vi "Main.vi"(11 "Module Admin":refnum<class "Delacor_lib_QMH_Cloneable Module Admin.lvclass">) -> ()   [LabVIEW 2024, in "Message.lvlib"]
doc: "This template is based off of the Queued Message Handler design pattern and the Queued Message Handler project template that ships with LabVIEW.\n\nThe main difference is that the queue is private to this module and communication between modules is performed via Broadcast and Request events.\n\nRequest events are wrapped in public API methods and are handled in the Event Handling Loop (EHL) of this VI. Any module can register for Broadcast events sent by this module. The EHL generates messages based on user interface actions.\n\nThe Message Handling Loop (MHL) processes messages generated by the EHL, or by other messages. The messages are string values, so new messages can be added easily to the Message Cases case structure in the MHL. Each message cluster can also provide an optional value for Message Data, which is a variant that can be converted to whatever message-specific data is required.\n_____\nBased on DQMH Dev Tools: Project Template 7.1.0.1503."
uses:
  Message.lvlib
  <vilib>/Delacor/Delacor QMH/Libraries/Cloneable Module Admin_class/Delacor_lib_QMH_Cloneable Module Admin.lvclass
  C:/Program Files (x86)/National Instruments/LabVIEW 2024/vi.lib/Delacor/Delacor QMH/Libraries/Module Admin_class/Delacor_lib_QMH_Module Admin.lvclass
  Module Data--cluster.ctl
  <vilib>/Delacor/Delacor QMH/Libraries/Cloneable Module Admin_class/Delacor_lib_QMH_Cloneable Module Admin.lvclass/Delacor_lib_QMH_Cloneable Module Admin.ctl
  Stop Argument--cluster.ctl
  <vilib>/Delacor/Delacor QMH/Libraries/Message Queue_class/Delacor_lib_QMH_Message Queue.lvclass/Delacor_lib_QMH_Message Queue.ctl
  <vilib>/Delacor/Delacor QMH/Libraries/Module Admin_class/Delacor_lib_QMH_Module Admin.lvclass/Delacor_lib_QMH_Module Admin.ctl
  Draw FP in Subpanel Argument--cluster.ctl
  Remove From Subpanel Argument--cluster.ctl
  Set Message Argument--cluster.ctl
  Append String Argument--cluster.ctl
  Set Text Font Settings Argument--cluster.ctl
  <vilib>/Utility/miscctls.llb/LVFontTypeDef.ctl
  <vilib>/Delacor/Delacor QMH/Libraries/Cloneable Module Admin_class/Delacor_lib_QMH_Get Module ID.vi
  <vilib>/Delacor/Delacor QMH/Libraries/Message Queue_class/Delacor_lib_QMH_Enqueue Message (Single).vi
  <vilib>/Delacor/Delacor QMH/Libraries/Module Admin_class/Delacor_lib_QMH_Get External Launch.vi
  <vilib>/Delacor/Delacor QMH/Libraries/Message Queue_class/Delacor_lib_QMH_Message Queue.lvclass
panel:
  out "Message":string
  out "error out":errorcluster
  out "String":string
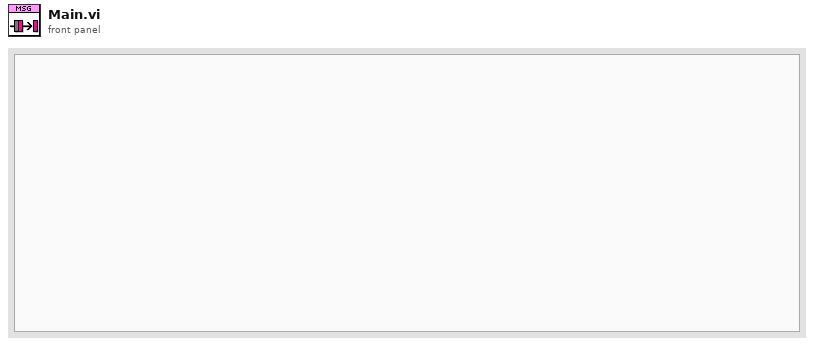
[diagram p1: front panel]
types:
  T1 = typedef "Message.lvlib/Request Events--cluster.ctl" = cluster{"Stop Module":refnum<user-event>, "Show Panel":refnum<user-event>, "Hide Panel":refnum<user-event>, "Show Diagram":refnum<user-event>, "Get Module Execution Status":refnum<user-event>, "Draw FP in Subpanel":refnum<user-event>, "Remove From Subpanel":refnum<user-event>, "Set Message":refnum<user-event>, "Append String":refnum<user-event>, "Set Text Font Settings":refnum<user-event>}
  T2 = typedef "Message.lvlib/Module Data--cluster.ctl" = cluster{"Status":string, "Sub Panel":refnum<vi>, "Message Ref":refnum<vi>}
  T3 = enum32{"invalid lock state", "Not Locked", "Locked (No Password)", "Password-protected"}
  T4 = typedef "Message.lvlib/Stop Argument--cluster.ctl" = cluster{"Module ID":i32, "Origin":string, "Exit via Stop Module Req?":bool, "Wait for Module to stop?":bool}
  T5 = typedef "Message.lvlib/Draw FP in Subpanel Argument--cluster.ctl" = cluster{"Module ID":i32, "Sub Panel":refnum<vi>}
  T6 = typedef "Message.lvlib/Remove From Subpanel Argument--cluster.ctl" = cluster{"Module ID":i32, "Boolean":bool}
  T7 = typedef "Message.lvlib/Set Message Argument--cluster.ctl" = cluster{"Module ID":i32, "Message":string}
  T8 = typedef "Message.lvlib/Append String Argument--cluster.ctl" = cluster{"Module ID":i32, "String":string}
  T9 = typedef "Message.lvlib/Set Text Font Settings Argument--cluster.ctl" = cluster{"Module ID":i32, "Font Settings":cluster{"Text.Font":T10, "Text.Justification":enum16{"Left", "Center", "Right"}}}
  T10 = typedef "LVFontTypeDef.ctl" = cluster{"Font Name":string, "Size":u16, "Bold":bool, "Italic":bool, "Underline":bool, "Strikeout":bool, "Color":u32}
  T11 = enum32{"Invalid", "Standard", "Closed", "Hidden", "Minimized", "Maximized"}
  T12 = cluster{"Text.Font":T10, "Text.Justification":enum16{"Left", "Center", "Right"}}
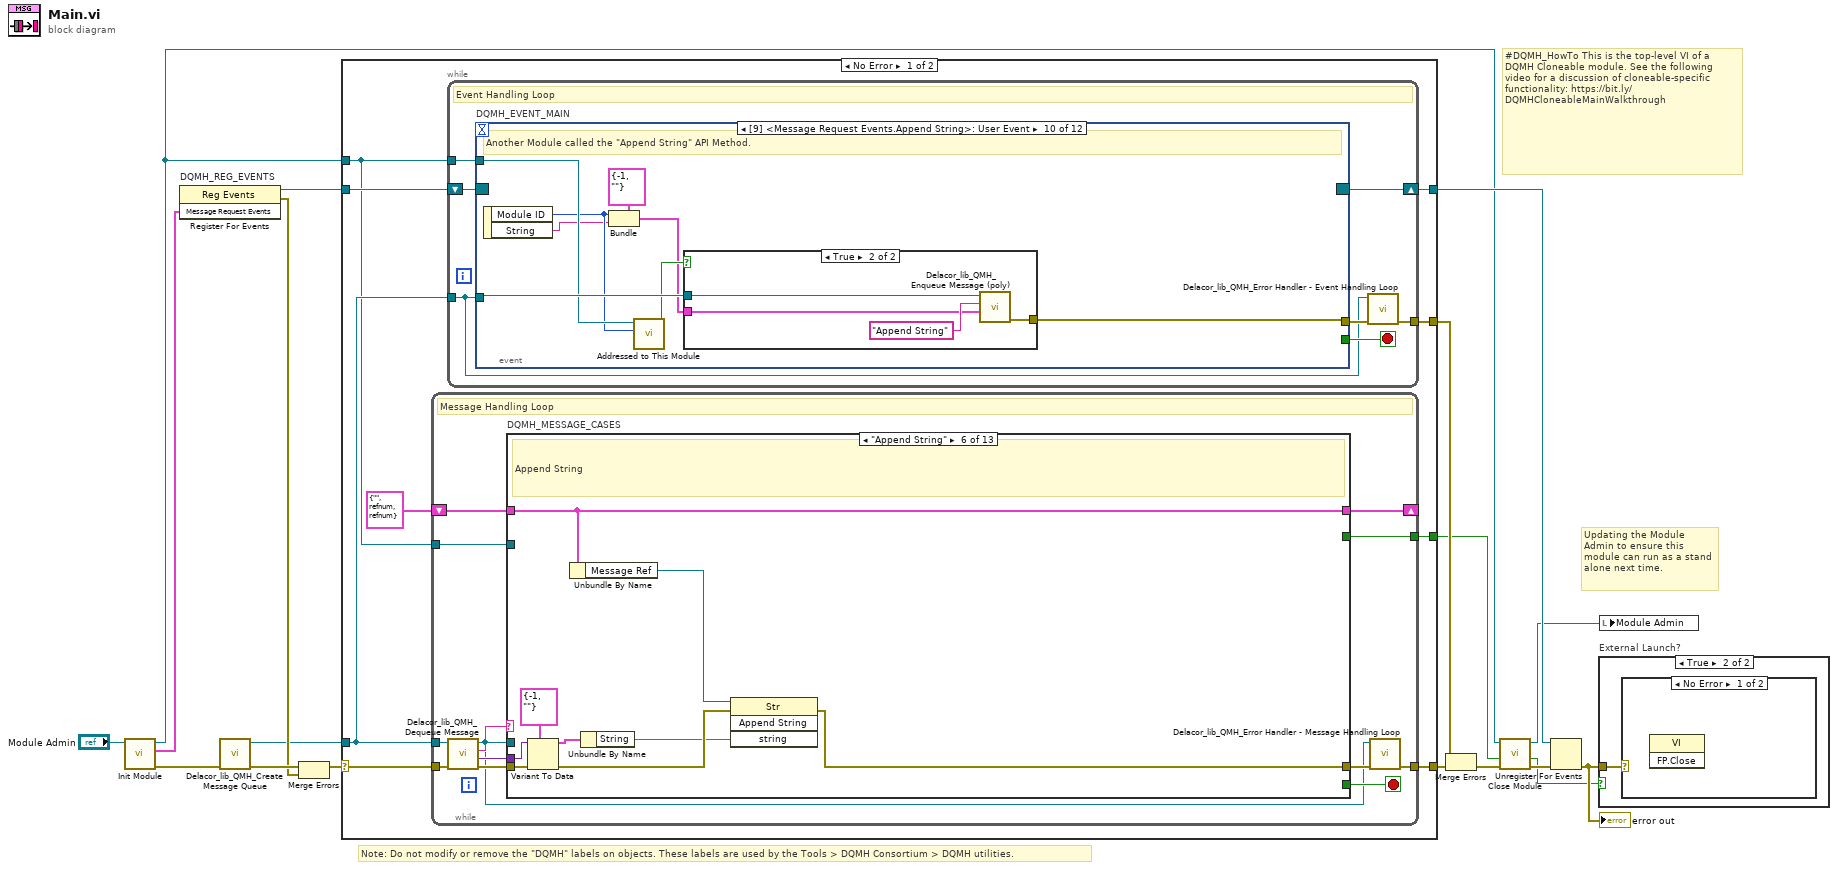
[diagram p0: block diagram]
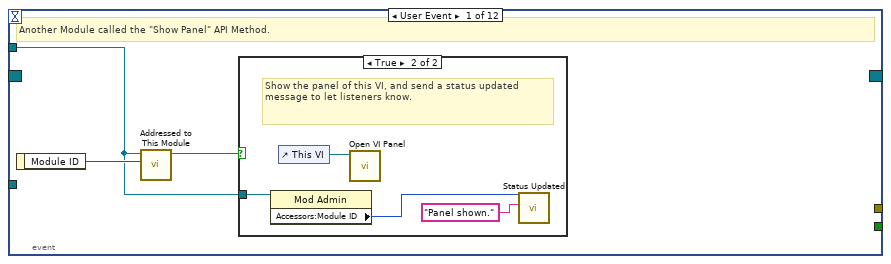
[diagram p2: hidden frame]
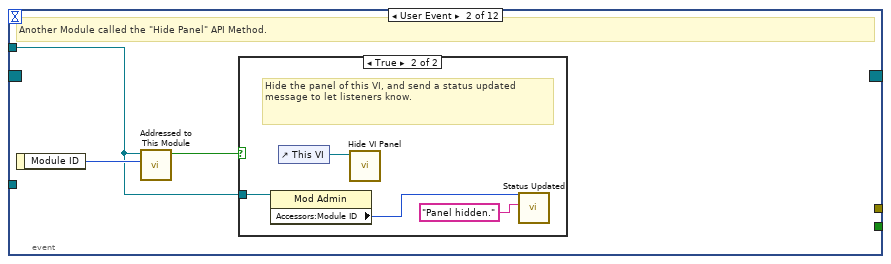
[diagram p4: hidden frame]
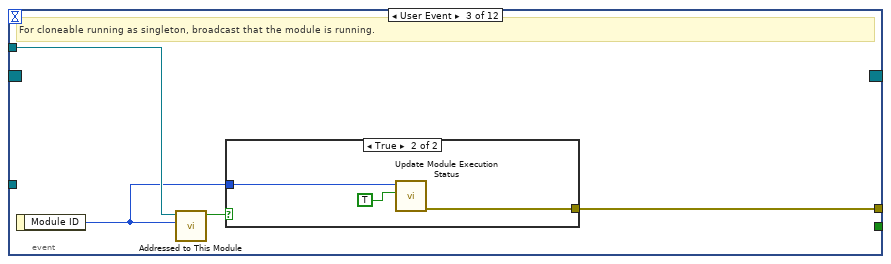
[diagram p6: hidden frame]
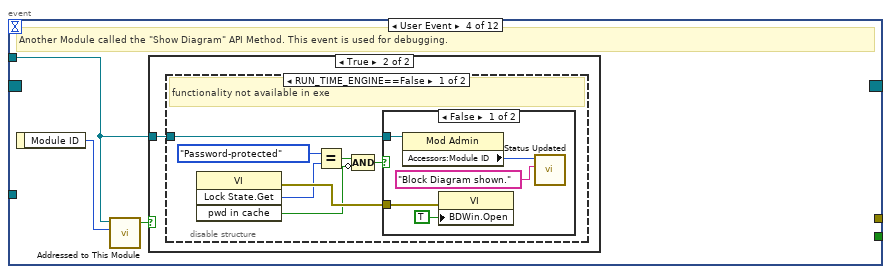
[diagram p8: hidden frame]
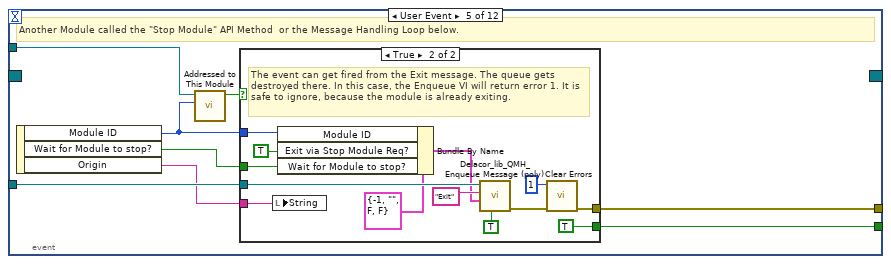
[diagram p12: hidden frame]
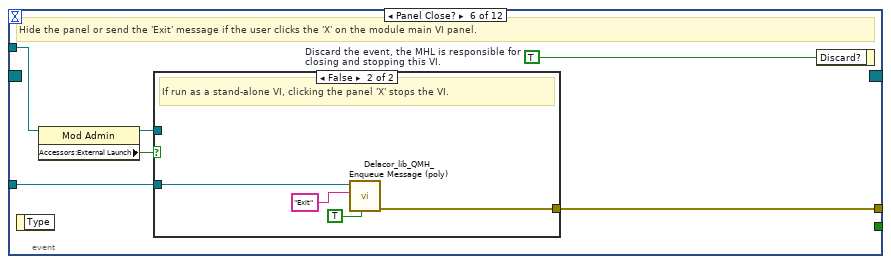
[diagram p14: hidden frame]
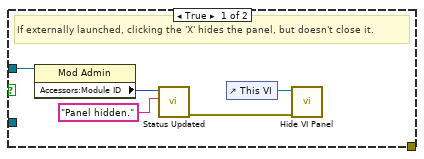
[diagram p15: hidden frame]
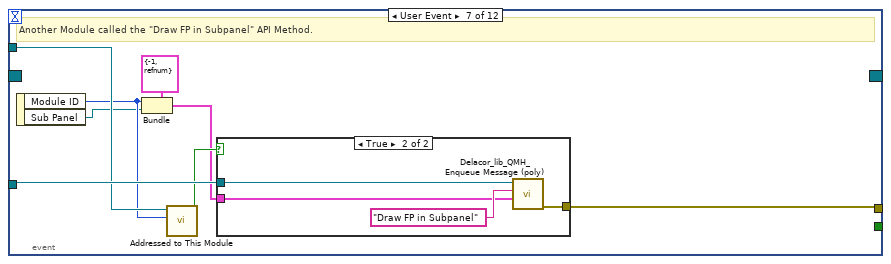
[diagram p16: hidden frame]
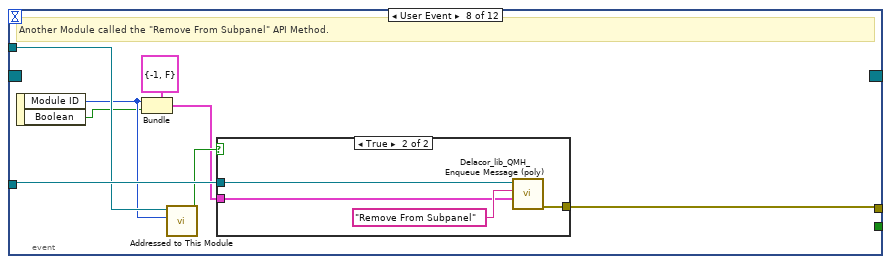
[diagram p18: hidden frame]
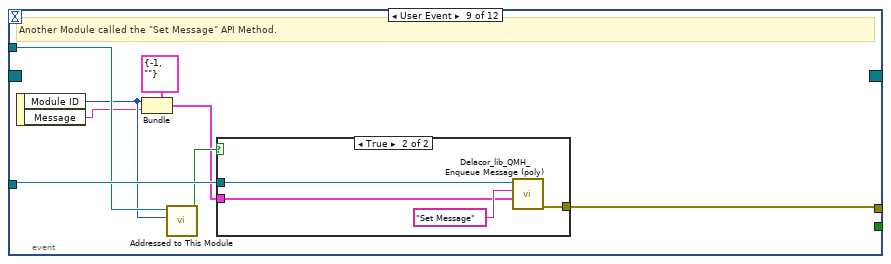
[diagram p20: hidden frame]
diagram:
  # "#DQMH_HowTo This is the top-level VI of a DQMH Cloneable module. See the following video for a discussion of cloneable-specific functionality: https://bit.ly/DQMHCloneableMainWalkthrough"
  # "Note: Do not modify or remove the \"DQMH\" labels on objects. These labels are used by the Tools > DQMH Consortium > DQMH utilities."
  # "Updating the Module Admin to ensure this module can run as a stand alone next time."
  n1 = call "Init Module.vi"("Cloneable Module Admin in"="Module Admin") -> ("error out"=w15:errorcluster, "Message Request Events"=w7:T1, "Cloneable Module Admin out"=w4:refnum<class "Delacor_lib_QMH_Cloneable Module Admin.lvclass">)  [unwired: 8 in]
  n2 = register-events "DQMH_REG_EVENTS"(w7) -> (reference out=w8:refnum<event-registration>, error out=w10:errorcluster)  [unwired: 2 in]
  n3 = call <vilib>:"Delacor_lib_QMH_Create Message Queue.vi"("error in"=w15) -> ("error out"=w12:errorcluster, "Message Queue"=w6:refnum<class "Delacor_lib_QMH_Message Queue.lvclass">)  [unwired: 9 in]
  n4 = Merge Errors(w12, w10) -> (w11:errorcluster)
  n5 = case shown="No Error" w11 {
    selector: w11 -> [w25 w358]
    tunnel: [w27 w357] -> w16
    tunnel: [w24 w356] -> w9
    tunnel: w8 -> [w22 w356]
    tunnel: w6 -> [w21 w349]
    tunnel: [w26 _] -> w17
    tunnel: w4 -> [w20 w352]
    tunnel: [w19 _] -> w2
    frame No Error {
      n6 = while {
        tunnel: w21 -> [w172]
        shift-right: [w179] -> _
        shift-left: T2 {"Status"="", "Sub Panel"=refnum, "Message Ref"=refnum} ("Data Cluster") -> [w180]
        tunnel: w25 -> [w183]
        tunnel: [w181] -> w27
        tunnel: w20 -> [w174]
        tunnel: [w173] -> w19
        stop <- w178 stop-if-true
        # "Message Handling Loop"
        n7 = call-dynamic "Delacor_lib_QMH_Dequeue Message.vi"("error in"=w183, "Message Queue in"=w172) -> ("error out"=w182:errorcluster, "Message Data"=w176:variant, "Message"=w177:string, "Message Queue out"=w175:refnum<class "Delacor_lib_QMH_Message Queue.lvclass">)  [unwired: 6 in]
        n8 = case "DQMH_MESSAGE_CASES" shown="\"Append String\"" w177 {
          selector: w177 -> [_ _ _ _ _ _ _ _ _ _ _ _ w338]
          tunnel: w175 -> [_ _ _ _ _ _ _ _ _ _ w302 w330 _]
          tunnel: w182 -> [w203 w207 w226 w246 w263 w272 w282 w291 w298 w300 w312 w336 w347]
          tunnel: [w201 w207 w222 w244 w262 w265 w275 w287 w297 w300 w308 w331 w348] -> w184
          tunnel: w180 -> [w194 w206 w212 w238 w261 w268 w277 w289 w296 w299 w306 w320 w345]
          tunnel: [w193 w206 w213 w234 w261 w268 w277 w289 w296 w299 w306 w320 w345] -> w179
          tunnel: [_ _ _ _ _ _ _ _ _ _ _ w329 _] -> w178
          tunnel: w176 -> [_ _ w221 w243 w260 w271 w281 w290 _ _ w305 w327 _]
          tunnel: w174 -> [w189 _ w210 w237 w257 _ _ _ _ _ w304 w322 w344]
          tunnel: [_ _ _ _ _ _ _ _ _ _ _ w325 _] -> w173
          frame "Initialize" {
            w186 = "Initial Message" ("Initial Message")
            # "Initialize - Any operation that needs to be done before the module can receive messages. Synchronize Caller Events.vi will inform Start Module.vi that the module has launched and is ready to receive messages. Module Did Init.vi will broadcast that the module initialized."
            n9 = call "Synchronize Caller Events.vi"("error in"=w203, "Module Admin"=w189) -> ("error out"=w202:errorcluster, "Module Admin out"=w188:refnum<class "Delacor_lib_QMH_Cloneable Module Admin.lvclass">)  [unwired: 8 in]
            n10 = property on="Property Node" class="Mod Admin"(reference=w188) -> ("Accessors:Module ID"=w187:i32, "Accessors:External Launch"=w190:bool)  [unwired: 1 in, 2 out]
            n11 = call "Module Name--constant.vi"("Module ID"=w187) -> ("Module Name"=w198:string)  [unwired: 10 in]
            n12 = property on="Property Node" class="VI"("Front Panel.Title"=w198) -> (reference out=w200:refnum<vi>, error out=w205:errorcluster)  [unwired: 2 in]
            n13 = Select(t=T11."Hidden" ("State"), s=w190, f=T11."Standard" ("State")) -> (s? t:f=w195:T11)
            n14 = control-ref of="Message"() -> (w185:refnum<vi>)
            n15 = invoke on="Invoke Node" class="VI" method="FP.Open"(reference=w200, error in=w205, "State"=w195) -> (reference out=w199:refnum<vi>, error out=w204:errorcluster)  [unwired: 2 in, 3 out]
            n16 = Bundle By Name(cluster=w194, "Status"=w186, "Message Ref"=w185) -> (w193:T2)
            n17 = invoke on="Invoke Node" class="VI" method="FP.Center"(reference=w199, error in=w204) -> ()  [unwired: 1 in, 3 out]
            n18 = call "Module Name--constant.vi"("Module ID"=w187) -> ("Module Name"=w191:string)  [unwired: 10 in]
            n19 = call "Module Did Init.vi"("error in"=w202, "Initialized?"=TRUE, "Origin"=w191, "Module ID"=w187) -> ("error out"=w201:errorcluster)  [unwired: 7 in]
            "String" <- w186
          }
          frame "---Module Specific---" {
            # "Separator -- The following cases handle messages specific to this Module."
          }
          frame "Draw FP in Subpanel" {
            # "Draw FP in Subpanel"
            n20 = Variant To Data(error in=w226, type=T5 {"Module ID"=-1, "Sub Panel"=refnum} ("Draw FP in Subpanel Argument"), Variant=w221) -> (data=w219:T5, error out=w223:errorcluster)
            n21 = property class="Mod Admin"(reference=w210) -> ("Accessors:Module ID"=w209:i32)  [unwired: 1 in, 2 out]
            n22 = Unbundle By Name(w219) -> ("Sub Panel"=w211:refnum<vi>)
            n23 = control-ref of="This VI"() -> (w216:refnum<vi>)
            n24 = property class="VI"(reference=w216, error in=w223) -> (reference out=w215:refnum<vi>, error out=w224:errorcluster, "FP.State"=w214:T11)
            n25 = case shown="\"Closed\"" w214 {
              tunnel: [w227 w230] -> w217
              tunnel: [w228 w232] -> w225
              tunnel: w224 -> [w228 w231]
              tunnel: w215 -> [w227 w229]
              frame "Closed" {
              }
              frame "Standard", Default {
                n26 = invoke class="VI" method="FP.Close"(reference=w229, error in=w231) -> (reference out=w230:refnum<vi>, error out=w232:errorcluster)  [unwired: 1 in, 1 out]
              }
            }
            n27 = invoke class="SubPnl" method="Insert VI"(reference=w211, error in=w225, "VI Ref"=w217) -> (reference out=w218:refnum<vi>, error out=w222:errorcluster)  [unwired: 1 in, 2 out]
            n28 = call "Status Updated.vi"("error in"=w222, "Status"="Front Panel Inserted in Subpanel", "Module ID"=w209) -> ()  [unwired: 8 in, 1 out]
            n29 = Bundle By Name(cluster=w212, "Sub Panel"=w218) -> (w213:T2)
          }
          frame "Remove From Subpanel" {
            # "Remove From Subpanel"
            n30 = Variant To Data(error in=w246, type=T6 {"Module ID"=-1, "Boolean"=FALSE} ("Remove From Subpanel Argument"), Variant=w243) -> (data=w241:T6, error out=w245:errorcluster)
            n31 = Unbundle By Name(w241) -> ()  [unwired: 2 out]
            n32 = property class="Mod Admin"(reference=w237) -> ("Accessors:Module ID"=w236:i32)  [unwired: 1 in, 2 out]
            n33 = Unbundle By Name(w238) -> ("Sub Panel"=w240:refnum<vi>)
            n34 = Not A Number/Path/Refnum?(number/path/refnum=w240) -> (NaN/Path/Refnum?=w239:bool)
            n35 = case shown="False" w239 {
              tunnel: w245 -> [w250 w252]
              tunnel: [w249 w252] -> w244
              tunnel: w240 -> [w248 _]
              tunnel: ["Panel Removed from Subpanel" "This module has not been inserted into the subpanel"] -> w235
              frame False {
                n36 = invoke class="SubPnl" method="Remove VI"(reference=w248, error in=w250) -> (error out=w249:errorcluster)  [unwired: 1 in, 2 out]
              }
              frame True {
              }
            }
            n37 = Bundle By Name(cluster=w238, "Sub Panel"=refnum<vi> refnum) -> (w234:T2)
            n38 = call "Status Updated.vi"("error in"=w244, "Status"=w235, "Module ID"=w236) -> ()  [unwired: 8 in, 1 out]
          }
          frame "Set Message" {
            # "Set Message"
            n39 = Variant To Data(error in=w263, type=T7 {"Module ID"=-1, "Message"=""} ("Set Message Argument"), Variant=w260) -> (data=w258:T7, error out=w262:errorcluster)
            n40 = Unbundle By Name(w258) -> ("Message"=w255:string)  [unwired: 1 out]
            "Message" <- w255
            n41 = property class="Mod Admin"(reference=w257) -> ("Accessors:Module ID"=w256:i32)  [unwired: 1 in, 2 out]
            n42 = Format Into String(format string="Message Set to: %s", w255) -> (resulting string=w254:string)  [unwired: 2 in, 1 out]
            n43 = call "Status Updated.vi"("Status"=w254, "Module ID"=w256) -> ()  [unwired: 9 in, 1 out]
          }
          frame "Append String" {
            # "Append String"
            n44 = Variant To Data(error in=w272, type=T8 {"Module ID"=-1, "String"=""} ("Append String Argument"), Variant=w271) -> (data=w269:T8, error out=w266:errorcluster)
            n45 = Unbundle By Name(w268) -> ("Message Ref"=w267:refnum<vi>)
            n46 = Unbundle By Name(w269) -> ("String"=w264:string)
            n47 = invoke class="Str" method="Append String"(reference=w267, error in=w266, "string"=w264) -> (error out=w265:errorcluster)  [unwired: 1 in, 3 out]
          }
          frame "Set Text Font Settings" {
            # "Set Text Font Settings"
            n48 = Variant To Data(error in=w282, type=T9 {"Module ID"=-1, "Font Settings"={"Text.Font"={"Font Name"="", "Size"=0, "Bold"=FALSE, "Italic"=FALSE, "Underline"=FALSE, "Strikeout"=FALSE, "Color"=0}, "Text.Justification"=enum."Left"}} ("Set Text Font Settings Argument"), Variant=w281) -> (data=w279:T9, error out=w276:errorcluster)
            n49 = Unbundle By Name(w277) -> ("Message Ref"=w274:refnum<vi>)
            n50 = Unbundle By Name(w279) -> ("Font Settings.Text.Font"=w278:T10, "Font Settings.Text.Justification"=w273:enum16{"Left", "Center", "Right"})
            n51 = property class="Str"(reference=w274, error in=w276, "Text.Font"=w278, "Text.Justify"=w273) -> (error out=w275:errorcluster)  [unwired: 1 out]
          }
          frame "Set Display Mode" {
            # "Set Display Mode"
            n52 = Variant To Data(error in=w291, type="", Variant=w290) -> (data=w283:string, error out=w288:errorcluster)
            n53 = Unbundle By Name(w289) -> ("Message Ref"=w286:refnum<vi>)
            n54 = case shown="\"Codes\"" w283 {
              tunnel: [u32 0 ("Display Style") u32 2 ("Display Style") u32 3 ("Display Style") u32 1 ("Display Style")] -> w284
              frame "Normal", Default {
              }
              frame "Password" {
              }
              frame "Hexadecimal" {
              }
              frame "Codes" {
              }
            }
            n55 = property class="Str"(reference=w286, error in=w288, "Display Style"=w284) -> (error out=w287:errorcluster)  [unwired: 1 out]
          }
          frame "---Copy This Frame---" {
            # "Duplicate this frame when creating new messages.  Change this comment in the duplicated frame to describe this message."
            n56 = Merge Errors(w298) -> (w297:errorcluster)
          }
          frame "---Exit and Error Handling---" {
            # "Separator - the following cases handle errors and exit messages."
          }
          frame "Error" {
            # "#DQMH_CodeRecommended - If the module is running in standalone mode (External Launch = FALSE), this code will pop up an error dialog and call the 'Exit' message if an error occurs. Add more fine-grained error management here."
            # "Error - Check the error message data and respond accordingly. This message is sent by the \"Error Handler\" VIs at the end of each loop in this application."
            n57 = property on="Property Node" class="Mod Admin"(reference=w304) -> ("Accessors:External Launch"=w303:bool, "Accessors:Module ID"=w301:i32)  [unwired: 1 in, 2 out]
            n58 = Variant To Data(error in=w312, type=errorcluster {"status"=FALSE, "code"=0, "source"=""} ("error constant"), Variant=w305) -> (data=w307:errorcluster, error out=w310:errorcluster)
            n59 = local write "error out"(w307) -> ()
            n60 = call "Error Reported.vi"("Error"=w307, "Module ID"=w301) -> ()  [unwired: 9 in, 1 out]
            n61 = case shown="False" w303 {
              tunnel: [w317 _] -> w309
              tunnel: w302 -> [w315 _]
              tunnel: w307 -> [w316 _]
              frame False {
                n62 = disable-structure shown="Default" {
                  disable-tunnel: w316 -> [w318 _]
                  frame condition #0 (active) {
                    # "If the module is running standalone, then pop up an error dialog and call the \"Exit\" message."
                    n63 = call <vilib>:"Simple Error Handler.vi"("error in (no error)"=w318) -> ()  [unwired: 4 in, 5 out]
                  }
                  frame condition #1 {
                    # "To prevent the Simple Error Handler VI from being loaded (e.g. when deploying to a Real-Time target), add the Conditional Disable Symbol \"DQMH_Disable_SEH\" to your project and set it to TRUE."
                  }
                }
                n64 = call-poly <vilib>:"Delacor_lib_QMH_Enqueue Message (poly).vi"("Priority Message? (F)"=TRUE, "Message"="Exit", "Message Queue in"=w315) -> ("error out"=w317:errorcluster)  [unwired: 7 in, 1 out]
              }
              frame True {
                # "If the module was launched externally, calling the Error Reported broadcast VI is the only action performed by the \"Error\" message. The module's caller can then process the error appropriately."
              }
            }
            n65 = Merge Errors(w310, w309) -> (w308:errorcluster)
          }
          frame "Exit" {
            w328 = 91  # 91: not all Exit messages will have an argument
            w329 = TRUE  # Stop the VI
            # "Release the message queue reference"
            # "#DQMH_CodeNeeded - Add any required cleanup code here."
            # "Exit - Exit the application."
            n66 = Variant To Data(error in=w336, type=T4 {"Module ID"=-1, "Origin"="", "Exit via Stop Module Req?"=FALSE, "Wait for Module to stop?"=FALSE} ("Stop Argument"), Variant=w327) -> (data=w324:T4, error out=w332:errorcluster)
            n67 = call <vilib>:"Clear Errors.vi"("error in (no error)"=w332, "specific error code to clear (0: all)"=w328) -> ("error out"=w335:errorcluster)  [unwired: 4 in, 1 out]
            n68 = property on="Property Node" class="Mod Admin"(reference=w322) -> ("Accessors:Module ID"=w321:i32)  [unwired: 1 in, 2 out]
            n69 = control-ref of="This VI"() -> (w323:refnum<vi>)
            n70 = call-dynamic "Delacor_lib_QMH_Release Message Queue.vi"("error in"=w335, "Message Queue"=w330) -> ("error out"=w334:errorcluster)  [unwired: 9 in]
            n71 = call "Handle Exit.vi"("Stop Argument"=w324, "Module Admin in"=w322, "VI reference"=w323) -> ("error out"=w333:errorcluster, "Wait for Stop?"=w325:bool)  [unwired: 7 in]
            n72 = Merge Errors(w334, w333) -> (w331:errorcluster)
            n73 = Unbundle By Name(w320) -> ("Sub Panel"=w319:refnum<vi>)
            n74 = call "Error Reported.vi"("Error"=w331, "Module ID"=w321) -> ()  [unwired: 9 in, 1 out]
            n75 = invoke class="SubPnl" method="Remove VI"(reference=w319) -> ()  [unwired: 2 in, 3 out]
          }
          frame Default {
            # "'Default' case only runs if there is a message that isn't defined in any of the other cases.  Output a programming error."
            n76 = property on="Property Node" class="Mod Admin"(reference=w344) -> ("Accessors:Module ID"=w343:i32)  [unwired: 1 in, 2 out]
            n77 = call "Module Name--constant.vi"("Module ID"=w343) -> ("Module Name"=w337:string)  [unwired: 10 in]
            n78 = Format Into String(format string="The invalid message string \"%s\" was received in the Message Handling Loop for module \"%s\".", w338, w337) -> (resulting string=w340:string)  [unwired: 2 in, 1 out]
            n79 = call <vilib>:"Error Cluster From Error Code.vi"("show call chain? (False)"=TRUE, "error message (\"\")"=w340, "error code (0)"=1) -> ("error out"=w346:errorcluster)  [unwired: 6 in]
            n80 = Merge Errors(w347, w346) -> (w348:errorcluster)
          }
        }
        n81 = call-dynamic "Delacor_lib_QMH_Error Handler - Message Handling Loop.vi"("error in"=w184, "Message Queue in"=w175) -> ("dup error in"=w181:errorcluster)  [unwired: 8 in, 1 out]
      }
      n82 = while {
        tunnel: w21 -> [w28]
        shift-right: [w31] -> w24
        shift-left: w22 -> [w32]
        tunnel: [w33] -> w26
        tunnel: w20 -> [w29]
        stop <- w30 stop-if-true
        # "Event Handling Loop"
        n83 = event "DQMH_EVENT_MAIN" shown="[9] <Message Request Events.Append String>: User Event" {
          selector: w32 -> [_ _ _ _ _ _ _ _ _ _ _ _]
          dyn-events: [_ _ _ _ _ _ _ _ _ _ _ _] -> w31
          timeout: _ -> [_ _ _ _ _ _ _ _ _ _ _ _]
          tunnel: [_ _ _ _ w75 _ _ _ _ _ _ _] -> w30
          tunnel: w28 -> [_ _ _ _ w78 w95 w114 w126 w138 w151 w163 w171]
          tunnel: [_ _ w52 _ w79 w98 w115 w127 w139 w144 w156 w168] -> w34
          tunnel: w29 -> [w35 w42 w50 w56 w77 w96 w112 w124 w136 w149 w161 _]
          event User Event {
            # "Another Module called the \"Show Panel\" API Method."
            n84 = event-data() -> ("Module ID"=w36:i32)  [unwired: 1 in]
            n85 = call "Addressed to This Module.vi"("Module ID from Argument"=w36, "Module Admin"=w35) -> ("Addressed to this instance?"=w37:bool)  [unwired: 8 in, 1 out]
            n86 = case shown="True" w37 {
              tunnel: w35 -> [_ w39]
              frame False {
              }
              frame True {
                # "Show the panel of this VI, and send a status updated message to let listeners know."
                n87 = property on="Property Node" class="Mod Admin"(reference=w39) -> ("Accessors:Module ID"=w38:i32)  [unwired: 1 in, 2 out]
                n88 = control-ref of="This VI"() -> (w41:refnum<vi>)
                n89 = call "Open VI Panel.vi"("VI"=w41) -> ()  [unwired: 10 in, 1 out]
                n90 = call "Status Updated.vi"("Status"="Panel shown." ("format string"), "Module ID"=w38) -> ()  [unwired: 9 in, 1 out]
              }
            }
          }
          event User Event {
            # "Another Module called the \"Hide Panel\" API Method."
            n91 = event-data() -> ("Module ID"=w43:i32)  [unwired: 1 in]
            n92 = call "Addressed to This Module.vi"("Module ID from Argument"=w43, "Module Admin"=w42) -> ("Addressed to this instance?"=w44:bool)  [unwired: 8 in, 1 out]
            n93 = case shown="True" w44 {
              tunnel: w42 -> [_ w46]
              frame False {
              }
              frame True {
                # "Hide the panel of this VI, and send a status updated message to let listeners know."
                n94 = property on="Property Node" class="Mod Admin"(reference=w46) -> ("Accessors:Module ID"=w45:i32)  [unwired: 1 in, 2 out]
                n95 = control-ref of="This VI"() -> (w48:refnum<vi>)
                n96 = call "Hide VI Panel.vi"("VI"=w48) -> ()  [unwired: 10 in, 1 out]
                n97 = call "Status Updated.vi"("Status"="Panel hidden." ("format string"), "Module ID"=w45) -> ()  [unwired: 9 in, 1 out]
              }
            }
          }
          event User Event {
            # "For cloneable running as singleton, broadcast that the module is running."
            n98 = event-data() -> ("Module ID"=w49:i32)  [unwired: 1 in]
            n99 = call "Addressed to This Module.vi"("Module ID from Argument"=w49, "Module Admin"=w50) -> ("Addressed to this instance?"=w51:bool)  [unwired: 8 in, 1 out]
            n100 = case shown="True" w51 {
              tunnel: [_ w55] -> w52
              tunnel: w49 -> [_ w54]
              frame False {
              }
              frame True {
                n101 = call "Update Module Execution Status.vi"("Running?"=TRUE, "Module ID"=w54) -> ("error out"=w55:errorcluster)  [unwired: 9 in]
              }
            }
          }
          event User Event {
            # "Another Module called the \"Show Diagram\" API Method. This event is used for debugging."
            n102 = event-data() -> ("Module ID"=w57:i32)  [unwired: 1 in]
            n103 = call "Addressed to This Module.vi"("Module ID from Argument"=w57, "Module Admin"=w56) -> ("Addressed to this instance?"=w58:bool)  [unwired: 8 in, 1 out]
            n104 = case shown="True" w58 {
              tunnel: w56 -> [_ w59]
              frame False {
              }
              frame True {
                n105 = disable-structure shown="RUN_TIME_ENGINE==False" {
                  disable-tunnel: w59 -> [w60 _]
                  frame condition #0 (active) {
                    # "functionality not available in exe"
                    n106 = invoke on="Invoke Node" class="VI" method="Lock State.Get"() -> (error out=w66:errorcluster, "Get Lock State"=w65:T3, "pwd in cache"=w62:bool)  [unwired: 4 in, 1 out]
                    n107 = Equal?(x=T3."Password-protected", y=w65) -> (x = y?=w63:bool)
                    n108 = Compound Arithmetic op=AND(w63, invert w62) -> (w61:bool)
                    n109 = case shown="False" w61 {
                      tunnel: w66 -> [w71 _]
                      tunnel: w60 -> [w68 _]
                      frame False {
                        n110 = property on="Property Node" class="Mod Admin"(reference=w68) -> ("Accessors:Module ID"=w67:i32)  [unwired: 1 in, 2 out]
                        n111 = property on="Property Node" class="VI"(error in=w71, "BDWin.Open"=TRUE ("Block Diagram Window:Open")) -> ()  [unwired: 1 in, 2 out]
                        n112 = call "Status Updated.vi"("Status"="Block Diagram shown." ("format string"), "Module ID"=w67) -> ()  [unwired: 9 in, 1 out]
                      }
                      frame True {
                        # "Password-protected VI, and the password is not in the cache. Do not show the diagram."
                      }
                    }
                  }
                  frame condition #1 {
                  }
                }
              }
            }
          }
          event User Event {
            # "Another Module called the \"Stop Module\" API Method  or the Message Handling Loop below."
            n113 = event-data() -> ("Module ID"=w73:i32, "Wait for Module to stop?"=w74:bool, "Origin"=w72:string)  [unwired: 1 in]
            n114 = call "Addressed to This Module.vi"("Module ID from Argument"=w73, "Module Admin"=w77) -> ("Addressed to this instance?"=w76:bool)  [unwired: 8 in, 1 out]
            n115 = case shown="True" w76 {
              tunnel: [_ w91] -> w79
              tunnel: w78 -> [_ w87]
              tunnel: [_ TRUE] -> w75
              tunnel: w74 -> [_ w82]
              tunnel: w73 -> [_ w84]
              tunnel: w72 -> [_ w80]
              frame False {
              }
              frame True {
                # "The event can get fired from the Exit message. The queue gets destroyed there. In this case, the Enqueue VI will return error 1. It is safe to ignore, because the module is already exiting."
                n116 = local write "String"(w80) -> ()
                n117 = Bundle By Name(cluster=T4 {"Module ID"=-1, "Origin"="", "Exit via Stop Module Req?"=FALSE, "Wait for Module to stop?"=FALSE} ("Stop Argument"), "Module ID"=w84, "Exit via Stop Module Req?"=TRUE, "Wait for Module to stop?"=w82) -> (w81:T4)
                n118 = call-poly <vilib>:"Delacor_lib_QMH_Enqueue Message (poly).vi"("Priority Message? (F)"=TRUE, "Message Data"=w81, "Message"="Exit", "Message Queue in"=w87) -> ("error out"=w92:errorcluster)  [unwired: 6 in, 1 out]
                n119 = call <vilib>:"Clear Errors.vi"("error in (no error)"=w92, "specific error code to clear (0: all)"=1) -> ("error out"=w91:errorcluster)  [unwired: 4 in, 1 out]
              }
            }
          }
          event Panel Close? {
            w97 = TRUE  # Discard the event, the MHL is responsible for closing and stopping this VI.
            # "Hide the panel or send the 'Exit' message if the user clicks the 'X' on the module main VI panel."
            n120 = event-data() -> ()  [unwired: 1 in, 1 out]
            n121 = property on="Property Node" class="Mod Admin"(reference=w96) -> (reference out=w93:refnum<class "Delacor_lib_QMH_Cloneable Module Admin.lvclass">, "Accessors:External Launch"=w94:bool)  [unwired: 1 in, 1 out]
            n122 = case shown="False" w94 {
              tunnel: w95 -> [_ w106]
              tunnel: [_ w107] -> w98
              tunnel: w93 -> [w100 _]
              frame True {
                # "If externally launched, clicking the 'X' hides the panel, but doesn't close it."
                n123 = property on="Property Node" class="Mod Admin"(reference=w100) -> ("Accessors:Module ID"=w99:i32)  [unwired: 1 in, 2 out]
                n124 = call "Status Updated.vi"("Status"="Panel hidden." ("format string"), "Module ID"=w99) -> ("error out"=w103:errorcluster)  [unwired: 9 in]
                n125 = control-ref of="This VI"() -> (w102:refnum<vi>)
                n126 = call "Hide VI Panel.vi"("error in"=w103, "VI"=w102) -> ()  [unwired: 9 in, 1 out]
              }
              frame False {
                # "If run as a stand-alone VI, clicking the panel 'X' stops the VI."
                n127 = call-poly <vilib>:"Delacor_lib_QMH_Enqueue Message (poly).vi"("Priority Message? (F)"=TRUE, "Message"="Exit", "Message Queue in"=w106) -> ("error out"=w107:errorcluster)  [unwired: 7 in, 1 out]
              }
            }
            n128 = event-data ("Event Filter Node")("Discard?"=w97) -> ()  [unwired: 1 in, 1 out]
          }
          event User Event {
            # "Another Module called the \"Draw FP in Subpanel\" API Method."
            n129 = event-data() -> ("Module ID"=w109:i32, "Sub Panel"=w108:refnum<vi>)  [unwired: 1 in]
            n130 = Bundle(cluster=T5 {"Module ID"=-1, "Sub Panel"=refnum} ("Draw FP in Subpanel Argument"), "Module ID"=w109, "Sub Panel"=w108) -> (w110:T5)
            n131 = call "Addressed to This Module.vi"("Module ID from Argument"=w109, "Module Admin"=w112) -> ("Addressed to this instance?"=w113:bool)  [unwired: 8 in, 1 out]
            n132 = case shown="True" w113 {
              tunnel: w114 -> [_ w118]
              tunnel: w110 -> [_ w116]
              tunnel: [_ w119] -> w115
              frame False {
              }
              frame True {
                n133 = call-poly <vilib>:"Delacor_lib_QMH_Enqueue Message (poly).vi"("Message Data"=w116, "Message"="Draw FP in Subpanel", "Message Queue in"=w118) -> ("error out"=w119:errorcluster)  [unwired: 7 in, 1 out]
              }
            }
          }
          event User Event {
            # "Another Module called the \"Remove From Subpanel\" API Method."
            n134 = event-data() -> ("Module ID"=w121:i32, "Boolean"=w120:bool)  [unwired: 1 in]
            n135 = Bundle(cluster=T6 {"Module ID"=-1, "Boolean"=FALSE} ("Remove From Subpanel Argument"), "Module ID"=w121, "Boolean"=w120) -> (w122:T6)
            n136 = call "Addressed to This Module.vi"("Module ID from Argument"=w121, "Module Admin"=w124) -> ("Addressed to this instance?"=w125:bool)  [unwired: 8 in, 1 out]
            n137 = case shown="True" w125 {
              tunnel: w126 -> [_ w130]
              tunnel: w122 -> [_ w128]
              tunnel: [_ w131] -> w127
              frame False {
              }
              frame True {
                n138 = call-poly <vilib>:"Delacor_lib_QMH_Enqueue Message (poly).vi"("Message Data"=w128, "Message"="Remove From Subpanel", "Message Queue in"=w130) -> ("error out"=w131:errorcluster)  [unwired: 7 in, 1 out]
              }
            }
          }
          event User Event {
            # "Another Module called the \"Set Message\" API Method."
            n139 = event-data() -> ("Module ID"=w133:i32, "Message"=w132:string)  [unwired: 1 in]
            n140 = Bundle(cluster=T7 {"Module ID"=-1, "Message"=""} ("Set Message Argument"), "Module ID"=w133, "Message"=w132) -> (w134:T7)
            n141 = call "Addressed to This Module.vi"("Module ID from Argument"=w133, "Module Admin"=w136) -> ("Addressed to this instance?"=w137:bool)  [unwired: 8 in, 1 out]
            n142 = case shown="True" w137 {
              tunnel: w138 -> [_ w142]
              tunnel: w134 -> [_ w140]
              tunnel: [_ w143] -> w139
              frame False {
              }
              frame True {
                n143 = call-poly <vilib>:"Delacor_lib_QMH_Enqueue Message (poly).vi"("Message Data"=w140, "Message"="Set Message", "Message Queue in"=w142) -> ("error out"=w143:errorcluster)  [unwired: 7 in, 1 out]
              }
            }
          }
          event User Event {
            # "Another Module called the \"Append String\" API Method."
            n144 = event-data() -> ("Module ID"=w146:i32, "String"=w145:string)  [unwired: 1 in]
            n145 = Bundle(cluster=T8 {"Module ID"=-1, "String"=""} ("Append String Argument"), "Module ID"=w146, "String"=w145) -> (w147:T8)
            n146 = call "Addressed to This Module.vi"("Module ID from Argument"=w146, "Module Admin"=w149) -> ("Addressed to this instance?"=w150:bool)  [unwired: 8 in, 1 out]
            n147 = case shown="True" w150 {
              tunnel: w151 -> [_ w155]
              tunnel: w147 -> [_ w153]
              tunnel: [_ w152] -> w144
              frame False {
              }
              frame True {
                n148 = call-poly <vilib>:"Delacor_lib_QMH_Enqueue Message (poly).vi"("Message Data"=w153, "Message"="Append String", "Message Queue in"=w155) -> ("error out"=w152:errorcluster)  [unwired: 7 in, 1 out]
              }
            }
          }
          event User Event {
            # "Another Module called the \"Set Text Font Settings\" API Method."
            n149 = event-data() -> ("Module ID"=w158:i32, "Font Settings"=w157:T12)  [unwired: 1 in]
            n150 = Bundle(cluster=T9 {"Module ID"=-1, "Font Settings"={"Text.Font"={"Font Name"="", "Size"=0, "Bold"=FALSE, "Italic"=FALSE, "Underline"=FALSE, "Strikeout"=FALSE, "Color"=0}, "Text.Justification"=enum."Left"}} ("Set Text Font Settings Argument"), "Module ID"=w158, "Font Settings"=w157) -> (w159:T9)
            n151 = call "Addressed to This Module.vi"("Module ID from Argument"=w158, "Module Admin"=w161) -> ("Addressed to this instance?"=w162:bool)  [unwired: 8 in, 1 out]
            n152 = case shown="True" w162 {
              tunnel: w163 -> [_ w167]
              tunnel: w159 -> [_ w165]
              tunnel: [_ w164] -> w156
              frame False {
              }
              frame True {
                n153 = call-poly <vilib>:"Delacor_lib_QMH_Enqueue Message (poly).vi"("Message Data"=w165, "Message"="Set Text Font Settings", "Message Queue in"=w167) -> ("error out"=w164:errorcluster)  [unwired: 7 in, 1 out]
              }
            }
          }
          event "Message": Shortcut Menu Selection (User) {
            n154 = event-data() -> ("ItemTag"=w169:string)  [unwired: 1 in]
            n155 = call-poly <vilib>:"Delacor_lib_QMH_Enqueue Message (poly).vi"("Message Data"=w169, "Message"="Set Display Mode", "Message Queue in"=w171) -> ("error out"=w168:errorcluster)  [unwired: 7 in, 1 out]
          }
        }
        n156 = call-dynamic "Delacor_lib_QMH_Error Handler - Event Handling Loop.vi"("error in"=w34, "Message Queue in"=w28) -> ("dup error in"=w33:errorcluster)  [unwired: 8 in, 1 out]
      }
    }
    frame Error {
      n157 = call "Synchronize Caller Events.vi"("Module Admin"=w352) -> ("Module Admin out"=w351:refnum<class "Delacor_lib_QMH_Cloneable Module Admin.lvclass">)  [unwired: 9 in, 1 out]
      n158 = property on="Property Node" class="Mod Admin"(reference=w351) -> ("Accessors:Module ID"=w350:i32)  [unwired: 1 in, 2 out]
      n159 = call-dynamic "Delacor_lib_QMH_Release Message Queue.vi"("error in"=w358, "Message Queue"=w349) -> ("error out"=w357:errorcluster)  [unwired: 9 in]
      n160 = call "Module Name--constant.vi"("Module ID"=w350) -> ("Module Name"=w355:string)  [unwired: 10 in]
      n161 = Format Into String(format string="An error occurred during initialization. %s is no longer running.", w355) -> (resulting string=w353:string)  [unwired: 2 in, 1 out]
      n162 = call "Error Reported.vi"("Additional Information"=w353, "Error"=w357, "Module ID"=w350) -> ()  [unwired: 8 in, 1 out]
    }
  }
  n163 = Merge Errors(w17, w16) -> (w18:errorcluster)
  n164 = call "Close Module.vi"("error in"=w18, "Wait for stop?"=w2, "Module Admin in"=w4) -> ("error out"=w14:errorcluster, "External Launch"=w1:bool, "Module Admin out"=w3:refnum<class "Delacor_lib_QMH_Cloneable Module Admin.lvclass">)  [unwired: 6 in]
  n165 = Unregister For Events(event registration refnum=w9, error in=w14) -> (error out=w13:errorcluster)
  "error out" <- w13
  n166 = case "External Launch?" shown="True" w1 {
    tunnel: w13 -> [_ w359]
    frame False {
    }
    frame True {
      n167 = case shown="No Error" w359 {
        frame No Error {
          n168 = invoke class="VI" method="FP.Close"() -> ()  [unwired: 3 in, 3 out]
        }
        frame Error {
          n169 = disable-structure shown="Default" {
            frame condition #0 (active) {
              n170 = invoke class="VI" method="FP.Open"("Activate"=TRUE ("Activate?")) -> ()  [unwired: 4 in, 5 out]
            }
            frame condition #1 {
              # "Don't show panel on error if running inside a built EXE."
            }
          }
        }
      }
    }
  }
  n171 = local write "Module Admin"(w3) -> ()
